vi "ETH_5 Data.vi"(7 "Enum":enum16{"Read", "Write"}(ring), 8 "error in":errorcluster, 11 "Motor Feedback":T1={"Run ACK"=FALSE, "RDR"=0.0, "Sector"=0.0, "Halls Speed"=0.0, "Mode"=TRUE, "Voltage Speed"=0.0, "Direction"="", "IDC"=0.0, "Movable average"=0.0, "VDC"=0.0}) -> (0 "error out":errorcluster, 3 "Motor Feedback":T1={"Run ACK"=FALSE, "RDR"=0.0, "Sector"=0.0, "Halls Speed"=0.0, "Mode"=TRUE, "Voltage Speed"=0.0, "Direction"="", "IDC"=0.0, "Movable average"=0.0, "VDC"=0.0})   [LabVIEW 2022 SP3]
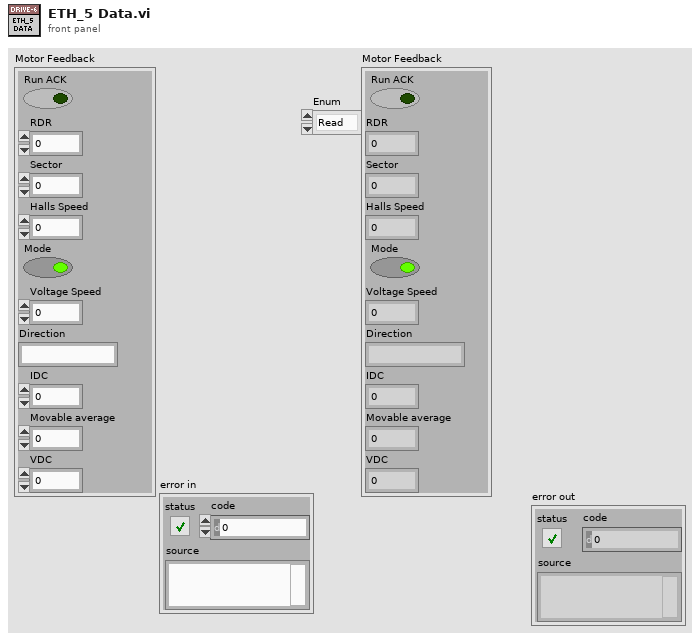
[diagram p1: front panel]
types:
  T1 = cluster{"Run ACK":bool, "RDR":dbl, "Sector":dbl, "Halls Speed":dbl, "Mode":bool, "Voltage Speed":dbl, "Direction":string, "IDC":dbl, "Movable average":dbl, "VDC":dbl}
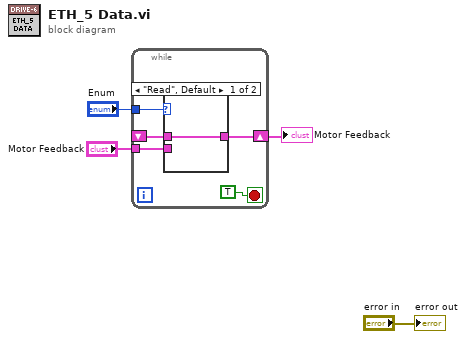
[diagram p0: block diagram]
diagram:
  n1 = while {
    tunnel: "Enum" -> [w9]
    tunnel: "Motor Feedback" -> [w7]
    shift-right: [w6] -> w1
    shift-left: _ -> [w5]
    stop <- TRUE stop-if-true
    n2 = case shown="\"Read\", Default" w9 {
      tunnel: w7 -> [_ w11]
      tunnel: [w10 w11] -> w6
      tunnel: w5 -> [w10 _]
      frame "Read", Default {
      }
      frame "Write" {
      }
    }
  }
  "Motor Feedback" <- w1
  "error out" <- "error in"
